vi "Write Center Point.vi"(10 "Center Point":dbl[unit], 11 "StartOpenLoopScan in":refnum<class "StartOpenLoopScan.lvclass">) -> (3 "StartOpenLoopScan out":refnum<class "StartOpenLoopScan.lvclass">)   [LabVIEW 2015, in "StartOpenLoopScan.lvclass"]
uses:
  StartOpenLoopScan.lvclass
  StartOpenLoopScan.lvclass/StartOpenLoopScan.ctl
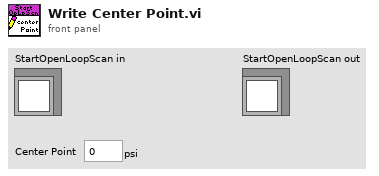
[diagram p1: front panel]
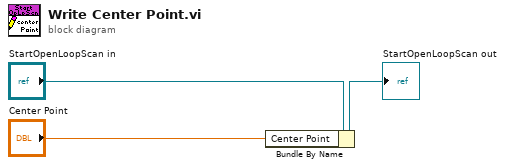
[diagram p0: block diagram]
diagram:
  n1 = Bundle By Name(cluster="StartOpenLoopScan in", "Center Point"="Center Point") -> (→"StartOpenLoopScan out":refnum<class "StartOpenLoopScan.lvclass">)
